vi "Websockets_Test No Connection Errors.vi"(8 "error in (no error)":errorcluster) -> (0 "error out":errorcluster)   [LabVIEW 2013]
uses:
  <vilib>/addons/_JKI Toolkits/Caraya/classes/Assert/Assert Equal Value_Variant.vi
  <vilib>/LabVIEW Open Source Project/MQTT Connection/MQTT_Connection/Connection/Connection.lvclass
  <vilib>/addons/_JKI Toolkits/Caraya/classes/Test/Test.lvclass
  <vilib>/addons/_JKI Toolkits/Caraya/classes/Assert/Assert.lvclass
  source/MQTT_Websockets/Connection/WebsocketsConnection.lvclass
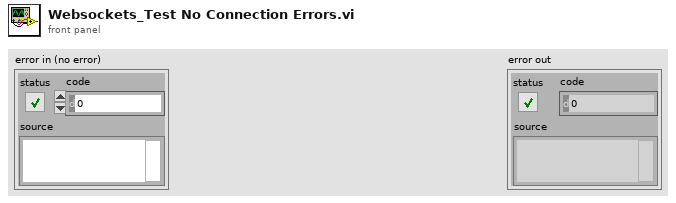
[diagram p1: front panel]
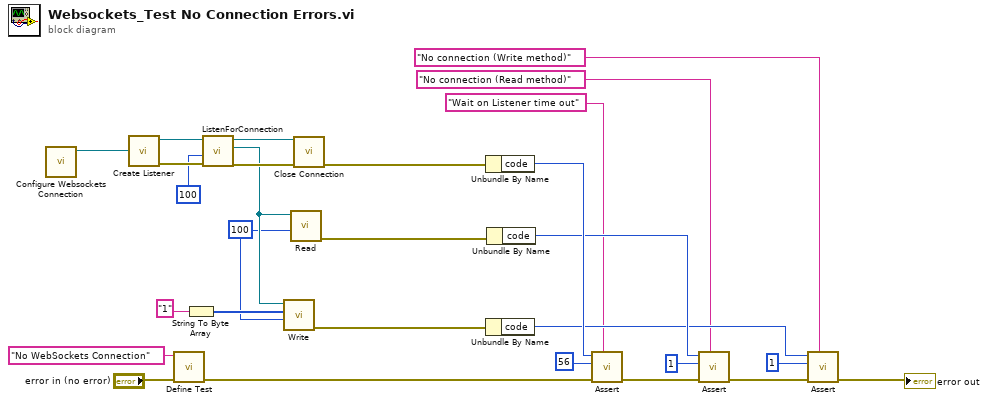
[diagram p0: block diagram]
diagram:
  w1 = 100 ("bytes to read")
  n1 = call "Configure Websockets Connection.vi"() -> ("WSConnection"=w4:refnum<class "WebsocketsConnection.lvclass">)  [unwired: 10 in, 1 out]
  n2 = call <vilib>:"Create Listener.vi"("Connection Configuration"=w4) -> ("error out"=w25:errorcluster, "Listener"=w28:refnum<class "Connection.lvclass">)  [unwired: 9 in]
  n3 = call <vilib>:"Define Test.vi"("error in (no error)"="error in (no error)", "Label (VI Title)"="No WebSockets Connection") -> ("error out"=w16:errorcluster)  [unwired: 9 in]
  n4 = String To Byte Array(string="1" ("data in")) -> (unsigned byte array=w23:u8[])
  n5 = call <vilib>:"ListenForConnection.vi"("error in (no error)"=w25, "timeout (2000 ms)"=100 ("timeout ms (wait forever: -1)"), "Listener"=w28) -> ("error out"=w26:errorcluster, "Connection"=w21:refnum<class "Connection.lvclass">, "Listener out"=w27:refnum<class "Connection.lvclass">)  [unwired: 5 in, 1 out]
  n6 = call <vilib>:"Write.vi"("timeout (2000 ms)"=w1, "Bytes"=w23, "Connection in"=w21) -> ("error out"=w19:errorcluster)  [unwired: 7 in, 1 out]
  n7 = call <vilib>:"Read.vi"("timeout (2000 ms)"=w1, "TCPConnection in"=w21) -> ("error out"=w18:errorcluster)  [unwired: 5 in, 4 out]
  n8 = call <vilib>:"Close Connection.vi"("error in (no error)"=w26, "Connection in"=w27) -> ("error out"=w20:errorcluster)  [unwired: 8 in, 1 out]
  n9 = Unbundle By Name(w20) -> ("code"=w15:i32)
  n10 = Unbundle By Name(w19) -> ("code"=w10:i32)
  n11 = Unbundle By Name(w18) -> ("code"=w11:i32)
  n12 = call-poly <vilib>:"Assert.vi"("Label"="Wait on Listener time out" ("Label (VI Title)"), "error in (no error)"=w16, "Y"=56 ("code"), "X"=w15) -> ("error out"=w13:errorcluster)  [unwired: 7 in]
  n13 = call-poly <vilib>:"Assert.vi"("Label"="No connection (Read method)" ("Label (VI Title)"), "error in (no error)"=w13, "Y"=1 ("code"), "X"=w11) -> ("error out"=w12:errorcluster)  [unwired: 7 in]
  n14 = call-poly <vilib>:"Assert.vi"("Label"="No connection (Write method)" ("Label (VI Title)"), "error in (no error)"=w12, "Y"=1 ("code"), "X"=w10) -> ("error out"=→"error out":errorcluster)  [unwired: 7 in]
